vi "Exemple_Metrics_Davies_Bouldin_Score.vi"() -> ()   [LabVIEW 2020]
uses:
  Objet/3 - Model selection and evaluation/3.3 - Metrics and scoring/davies_bouldin_score/Davies_Bouldin_Score.vi
panel:
  out "Score":string
  out "error out":errorcluster caption="sortie d'erreur"
  in  "error in (no error)":errorcluster caption="entrée d'erreur (pas d'erreur)"
  in  "labels":string[][](array[string])=[["0"], ["1"], ["1"]]
  in  "X":string[][](array[string])=[["0", "1"], ["2", "4"], ["6", "8"]]
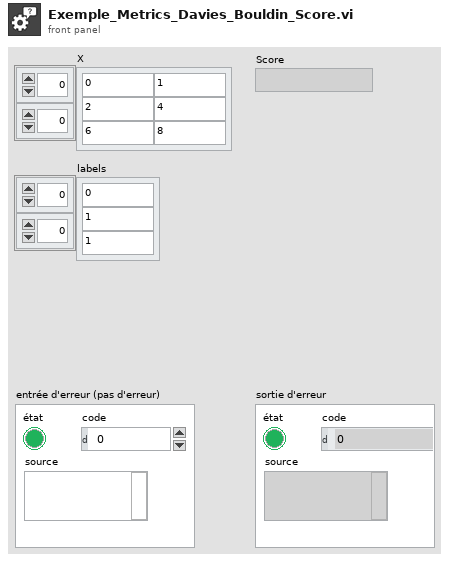
[diagram p1: front panel]
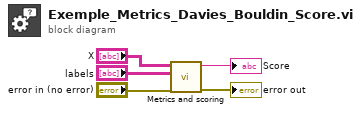
[diagram p0: block diagram]
diagram:
  n1 = call-poly "Metrics and scoring.vi"("error in (no error)"="error in (no error)", "labels"="labels", "X"="X") -> ("error out"=→"error out":errorcluster, "Score"=→"Score":string)  [unwired: 7 in]
